vi "Calibration_flt.vi"(11 "command line":string) -> (3 "Calibration Complete?":bool)   [LabVIEW 2017]
panel:
  out "x != y?":bool
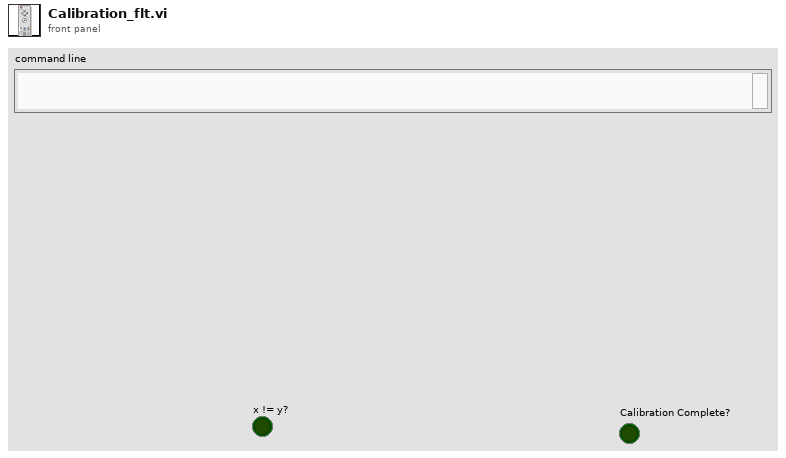
[diagram p1: front panel]
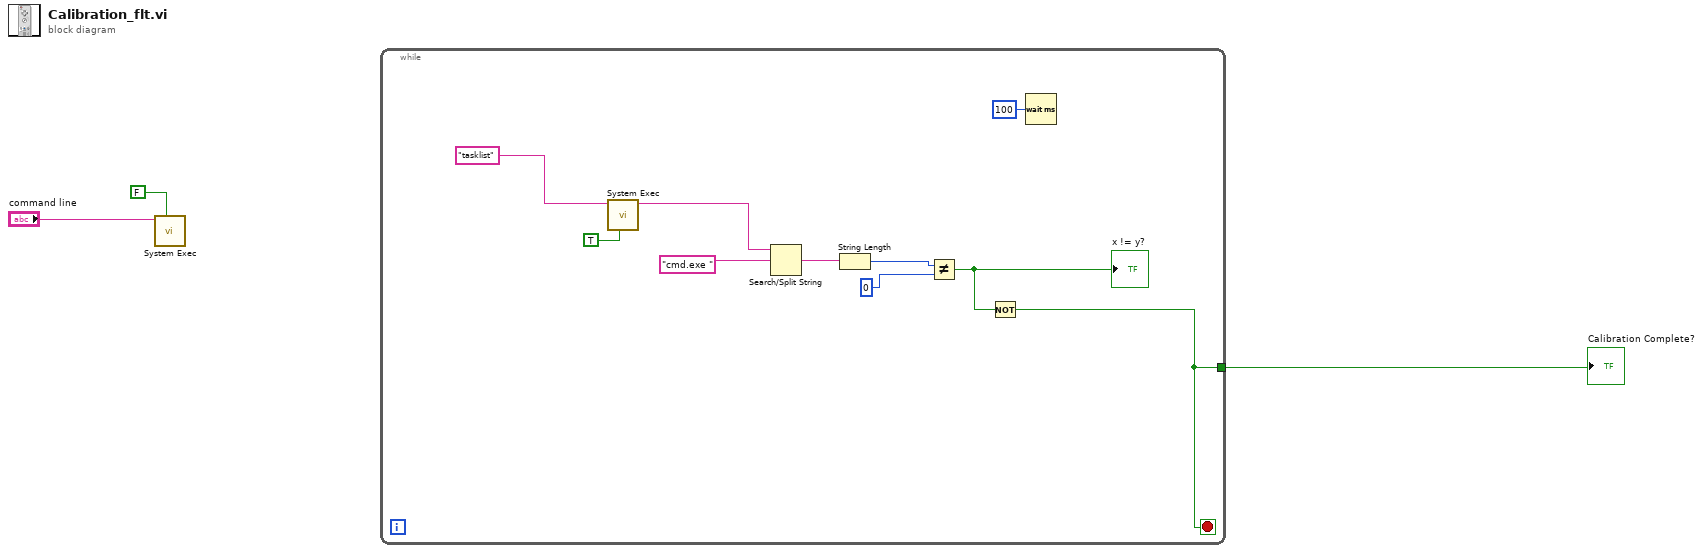
[diagram p0: block diagram]
diagram:
  n1 = call <vilib>:"System Exec.vi"("wait until completion? (T)"=FALSE, "command line"="command line") -> ()  [unwired: 6 in, 4 out]
  n2 = while {
    tunnel: [w4] -> w2
    stop <- w4 stop-if-true
    n3 = call <vilib>:"System Exec.vi"("run minimized? (F)"=TRUE, "command line"="tasklist") -> ("standard output"=w12:string)  [unwired: 6 in, 3 out]
    n4 = Search/Split String(string=w12, search string/char (-)="cmd.exe ") -> (match + rest of string=w10:string)  [unwired: 1 in, 2 out]
    n5 = String Length(string=w10) -> (length=w9:i32)
    n6 = Not Equal?(x=w9, y=0) -> (x != y?=w6:bool)
    "x != y?" <- w6
    n7 = Not(x=w6) -> (.not. x?=w4:bool)
    n8 = Wait (ms)(milliseconds to wait=u32 100) -> ()  [unwired: 1 out]
  }
  "Calibration Complete?" <- w2
